vi "AnyBuilderBegin.vi"(7 "error in":errorcluster) -> (0 "error out":errorcluster, 3 "Builder Ref Out":T1)   [LabVIEW 2019, in "grpc-lvsupport.lvlib"]
uses:
  grpc-lvsupport.lvlib
  Shared/grpcId.ctl
  <vilib>/Utility/error.llb/Error Cluster From Error Code.vi
  <resource>/labview_grpc_server.dll
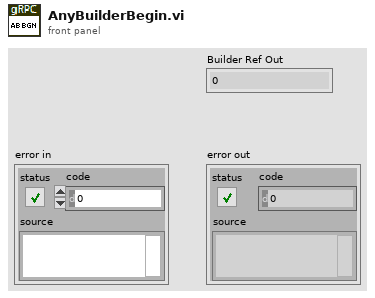
[diagram p1: front panel]
types:
  T1 = typedef "grpc-lvsupport.lvlib/grpcId.ctl" = u64
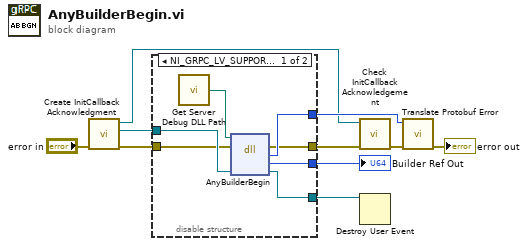
[diagram p0: block diagram]
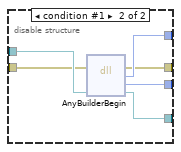
[diagram p2: hidden frame]
diagram:
  n1 = call "Create InitCallback Acknowledgment.vi"("error in (no error)"="error in") -> ("error out"=w6:errorcluster, "Init'd"=w8:refnum<user-event>, "InitCallbackAck Registration"=w5:refnum<event-registration>)  [unwired: 8 in]
  n2 = disable-structure shown="NI_GRPC_LV_SUPPORT_DEBUG==True&&RUN_TIME_ENGINE==False" {
    disable-tunnel: [w16 w23] -> w10
    disable-tunnel: [w15 w22] -> w9
    disable-tunnel: w8 -> [w14 w21]
    disable-tunnel: w6 -> [w13 w20]
    disable-tunnel: [w12 w19] -> w4
    disable-tunnel: [w11 w18] -> w2
    frame condition #0 (active) {
      n3 = call "Get Server Debug DLL Path.vi"() -> ("Server Debug DLL Path"=w17:path)
      n4 = dll-call lib="?" fn="AnyBuilderBegin"(path in=w17, error in=w13, "InitCallbacksAck"=w14) -> (error out=w12:errorcluster, "return type"=w15:i32, "anyId"=w16:u64, "InitCallbacksAck"=w11:refnum<user-event>)  [unwired: 2 in, 1 out]
    }
    frame condition #1 {
      n5 = dll-call lib="C:/Program Files (x86)/National Instruments/LabVIEW 2024/resource/labview_grpc_server.*" fn="AnyBuilderBegin"(error in=w20, "InitCallbacksAck"=w21) -> (error out=w19:errorcluster, "return type"=w22:i32, "anyId"=w23:u64, "InitCallbacksAck"=w18:refnum<user-event>)  [unwired: 3 in, 1 out]
    }
  }
  "Builder Ref Out" <- w10
  n6 = call "Check InitCallback Acknowledgement.vi"("error in (no error)"=w4, "InitCallbackAck Registration"=w5) -> ("error out"=w3:errorcluster)  [unwired: 9 in]
  n7 = Destroy User Event(user event=w2) -> ()  [unwired: 1 in, 1 out]
  n8 = call "Translate Protobuf Error.vi"("error in"=w3, "Error Code"=w9) -> ("error out"=→"error out":errorcluster)  [unwired: 9 in]
